vi "Encryption.U8 Array to Hex String.VI"(1 "U8 Array In":u8[](array[numeric])) -> (0 "Hex String":string)   [LabVIEW 2024, in "KATE_Lib.lvlib" / "Encryption.lvlib"]
uses:
  Encryption.lvlib
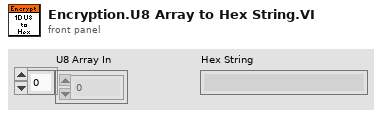
[diagram p1: front panel]
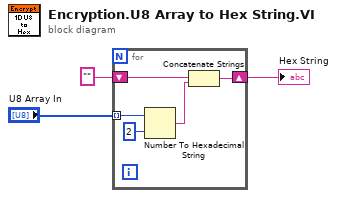
[diagram p0: block diagram]
diagram:
  n1 = for {
    tunnel: "U8 Array In" -> [w8] mode=indexing
    shift-right: [w5] -> w1
    shift-left: "" -> [w7]
    n2 = Number To Hexadecimal String(1:i16 2 ("width (-)"), 2:w8) -> (0:w6:string)
    n3 = Concatenate Strings(w7, w6) -> (w5:string)
  }
  "Hex String" <- w1
